vi "TestingPoint.vi"() -> ()   [LabVIEW 2016]
uses:
  <vilib>/Rock Robotics/WPI/Utilities/WPI_GetSetVariantRefNum.vi
panel:
  in  "Zero Yaw":bool
  in  "Config":T1={"Angle"=360.0, "MaxVelocity"=60.0, "MaxAccel"=50.0, "InitialVelocity"=0.0, "FinalVelocity"=0.0}
  out "Outputs":dbl(graph)
  in  "Go":bool
  in  "Go Backwards":bool
  out "Angular velocity":cluster{dbl, "vel":dbl}(graph)
  out "Angle":cluster{dbl, "pos":dbl}(graph)={50.0, "pos"=48.31556625}
  in  "Angular Constants":T2={"FF"=0.0066, "AFF"=0.0, "PID gains"={"P"=0.0, "I"=0.0, "D"=0.0}} {"PID gains"."D" format="%.3f"; "PID gains"."I" format="%.3f"; "PID gains"."P" format="%.3f"}
  # "MAKE DEFAULT"
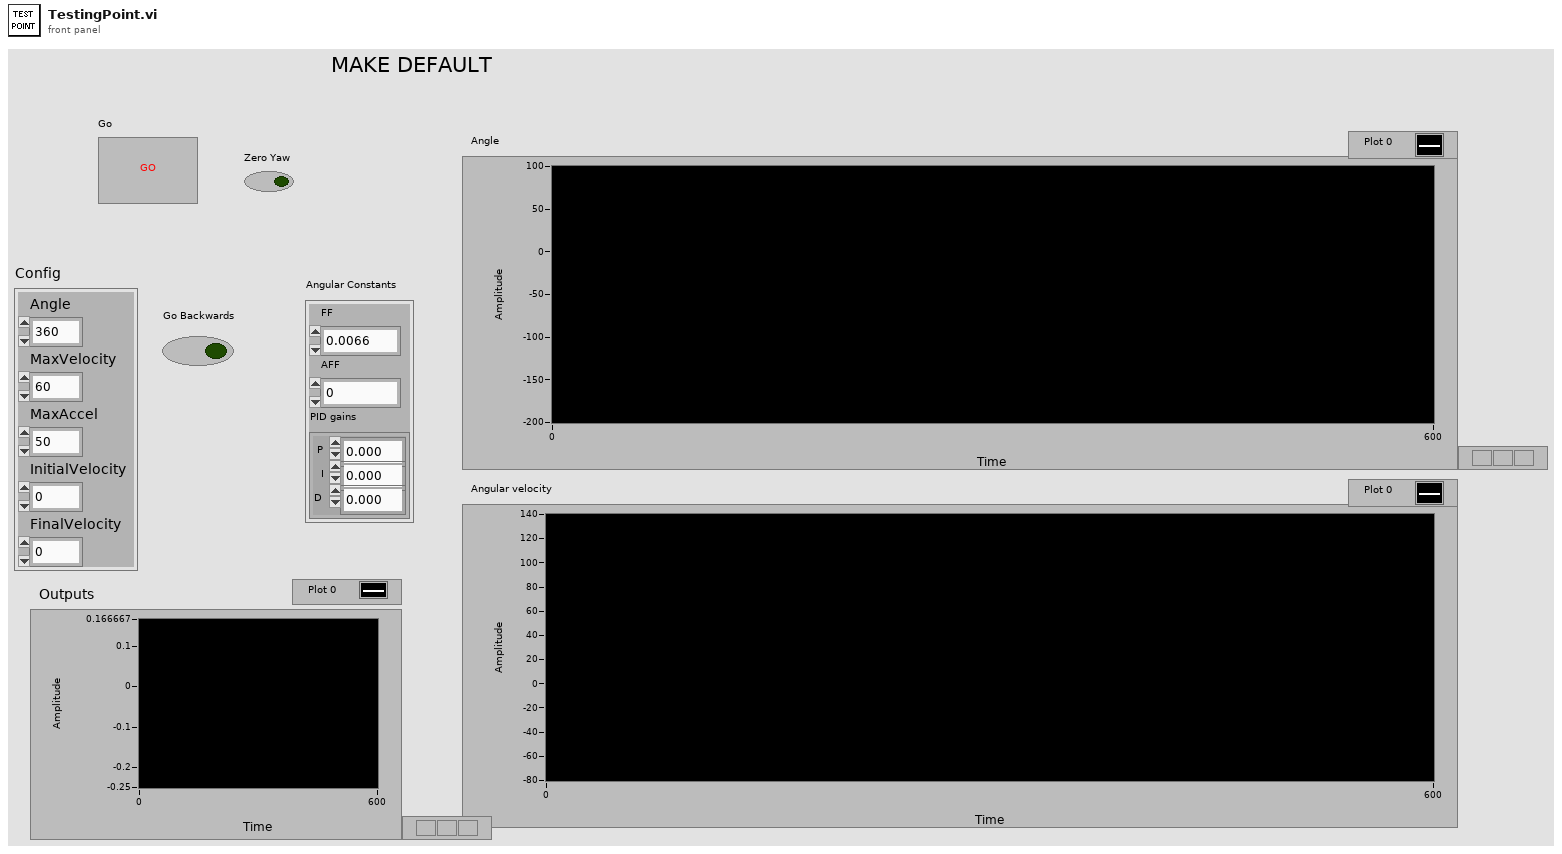
[diagram p1: front panel]
types:
  T1 = cluster{"Angle":dbl, "MaxVelocity":dbl, "MaxAccel":dbl, "InitialVelocity":dbl, "FinalVelocity":dbl}
  T2 = cluster{"FF":dbl, "AFF":dbl, "PID gains":cluster{"P":dbl, "I":dbl, "D":dbl}}
  T3 = cluster{"Yaw":dbl, "Roll":dbl, "Pitch":dbl, "Heading":dbl, "Fused Heading":dbl}
  T4 = typedef "WPI_RobotDriveDevRef.ctl" = cluster{"DevStatus":errorcluster, "Motors[]":T5[], "Square Inputs":bool, "Max Output":dbl}
  T5 = typedef "WPI_MotorControlDeviceRef.ctl" = cluster{"DeviceStatus":errorcluster, "Type":T6, "PWM":cluster{"PWM Channel":T7, "DeadBand":T8}, "CAN":cluster{"Device Number":u8, "SetOutput VI Ref":variant, "GetOutput VI Ref":variant, "Enable VI Ref":variant, "Disable VI Ref":variant, "Data":variant}, "Invert":bool}
  T6 = typedef "WPI_MotorControlType.ctl" = enum16{"PWM", "CAN"}
  T7 = typedef "FPGA_DIOPWMChannel.ctl" = enum8{"PWM 0", "PWM 1", "PWM 2", "PWM 3", "PWM 4", "PWM 5", "PWM 6", "PWM 7", "PWM 8", "PWM 9", "PWM MXP 0", "PWM MXP 1", "PWM MXP 2", "PWM MXP 3", "PWM MXP 4", "PWM MXP 5", "PWM MXP 6", "PWM MXP 7", "PWM MXP 8", "PWM MXP 9", "Invalid"}
  T8 = typedef "WPI_PWMDeadband.ctl" = cluster{"Name":string, "maxPositivePwm":i32, "minPositivePwm":i32, "centerPwm":i32, "maxNegativePwm":i32, "minNegativePwm":i32, "angularRange":u16}
  T9 = cluster{dbl, "distance/rotation":dbl, "distance/rotation":dbl}
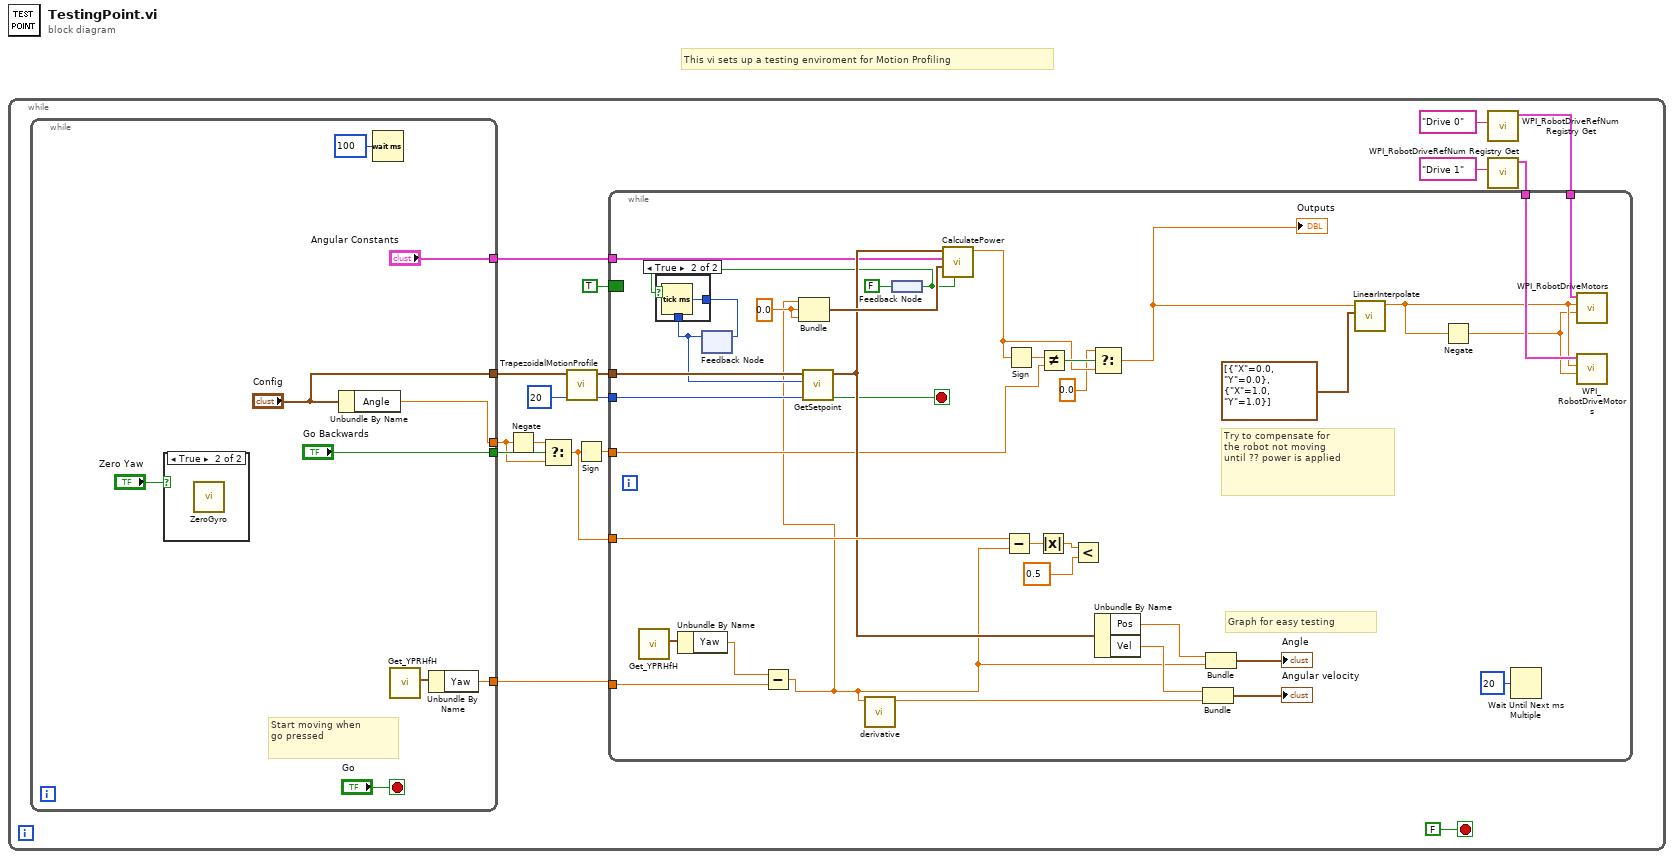
[diagram p0: block diagram]
diagram:
  # "This vi sets up a testing enviroment for Motion Profiling"
  n1 = while {
    stop <- FALSE stop-if-true
    n2 = while {
      tunnel: ["Go Backwards"] -> w7
      tunnel: [w23] -> w6
      tunnel: ["Config"] -> w5
      tunnel: ["Angular Constants"] -> w4
      tunnel: [w18] -> w1
      stop <- "Go" stop-if-true
      # "Start moving when\ngo pressed"
      n3 = case shown="True" "Zero Yaw" {
        frame False {
        }
        frame True {
          n4 = call "ZeroGyro.vi"() -> ()  [unwired: 11 in, 1 out]
        }
      }
      n5 = Unbundle By Name("Config") -> ("Angle"=w23:dbl)
      n6 = Wait (ms)(milliseconds to wait=u32 100 ("millisecond multiple")) -> ()  [unwired: 1 out]
      n7 = call <vilib>:"Get_YPRHfH.vi"() -> ("YRPHfH"=w19:T3)  [unwired: 11 in]
      n8 = Unbundle By Name(w19) -> ("Yaw"=w18:dbl)
    }
    n9 = Negate(x=w6) -> (-x=w16:dbl)
    n10 = Select(t=w16, s=w7, f=w6) -> (s? t:f=w9:dbl)
    n11 = call "TrapezoidalMotionProfile.vi"("dt"=u32 20, "Config"=w5) -> ("dt"=w12:u32, "Profile"=w17:cluster{"Pos":dbl, "Vel":dbl, "Accel":dbl}[])  [unwired: 8 in]
    n12 = Sign(1:w9) -> (0:w8:dbl)
    n13 = call <vilib>:"WPI_RobotDriveRefNum Registry Get.vi"("refnum name"="Drive 0") -> ("RobotDriveDevRef"=w3:T4)  [unwired: 9 in, 1 out]
    n14 = call <vilib>:"WPI_RobotDriveRefNum Registry Get.vi"("refnum name"="Drive 1") -> ("RobotDriveDevRef"=w2:T4)  [unwired: 9 in, 1 out]
    n15 = while {
      tunnel: w17 -> [w53]
      tunnel: w9 -> [w58]
      border: TRUE ("Reset") -> [_]
      tunnel: w12 -> [w52]
      tunnel: w8 -> [w44]
      tunnel: w4 -> [w40]
      tunnel: w3 -> [w37]
      tunnel: w2 -> [w36]
      tunnel: w1 -> [w31]
      stop <- w46 stop-if-true
      w55 = 0.0 ("distance/rotation")
      # "Try to compensate for\nthe robot not moving\nuntil ?? power is applied"
      # "Graph for easy testing"
      n16 = call <vilib>:"Get_YPRHfH.vi"() -> ("YRPHfH"=w33:T3)  [unwired: 11 in]
      n17 = Unbundle By Name(w33) -> ("Yaw"=w32:dbl)
      n18 = feedback #1() -> (w38:u32)  [unwired: 1 in]
      n19 = Subtract(x=w32, y=w31) -> (x-y=w27:dbl)
      n20 = Bundle(w27, "distance/rotation"=w55, "distance/rotation"=w55) -> (w56:T9)  [unwired: 1 in]
      n21 = call "GetSetpoint.vi"("dt"=w52, "Start Time"=w38, "Profile"=w53) -> ("Profile done?"=w46:bool, "Setpoints"=w51:cluster{"Pos":dbl, "Vel":dbl, "Accel":dbl})  [unwired: 7 in]
      n22 = call "derivative.vi"("x"=w27) -> ("dx/dt"=w57:dbl)  [unwired: 10 in]
      n23 = feedback-in #2(FALSE ("Reset")) -> ()
      n24 = feedback #2() -> (w34:bool)
      n25 = case shown="True" w34 {
        tunnel: [w63 w64] -> w39
        tunnel: w38 -> [w63 _]
        frame False {
        }
        frame True {
          n26 = Tick Count (ms)() -> (millisecond timer value=w64:u32)
        }
      }
      n27 = feedback-in #1(w39) -> ()
      n28 = call "CalculatePower.vi"("Reset"=w34, "Process Variables"=w56, "Constants"=w40, "Setpoints"=w51) -> ("Power"=w42:dbl)  [unwired: 7 in]
      n29 = Subtract(x=w58, y=w27) -> (x-y=w61:dbl)
      n30 = Sign(1:w42) -> (0:w45:dbl)
      n31 = Absolute Value(x=w61) -> (abs(x)=w60:dbl)
      n32 = Not Equal?(x=w45, y=w44) -> (x != y?=w43:bool)
      n33 = Less?(x=w60, y=0.5 ("Closeness at end")) -> ()  [unwired: 1 out]
      n34 = Select(t=0.0, s=w43, f=w42) -> (s? t:f=w30:dbl)
      "Outputs" <- w30
      n35 = Unbundle By Name(w51) -> ("Pos"=w50:dbl, "Vel"=w49:dbl)
      n36 = Bundle("Vel"=w49, "dx/dt"=w57) -> (→"Angular velocity":cluster{"Vel":dbl, "dx/dt":dbl})  [unwired: 1 in]
      n37 = Bundle("Pos"=w50, w27) -> (→"Angle":cluster{"Pos":dbl, dbl})  [unwired: 1 in]
      n38 = call "LinearInterpolate.vi"("Points"=cluster{"X":dbl, "Y":dbl}[] [{"X"=0.0, "Y"=0.0}, {"X"=1.0, "Y"=1.0}], "Value"=w30) -> ("Output"=w29:dbl)  [unwired: 9 in]
      n39 = Negate(x=w29) -> (-x=w28:dbl)
      n40 = Wait Until Next ms Multiple(millisecond multiple=u32 20) -> ()  [unwired: 1 out]
      n41 = call <vilib>:"WPI_RobotDriveMotors.vi"("RightSpeed"=w28, "LeftSpeed"=w29, "RobotDriveDevRef"=w37) -> ()  [unwired: 6 in, 3 out]
      n42 = call <vilib>:"WPI_RobotDriveMotors.vi"("RightSpeed"=w28, "LeftSpeed"=w29, "RobotDriveDevRef"=w36) -> ()  [unwired: 6 in, 3 out]
    }
  }
